vi "stringsubsect.vi"() -> ()   [LabVIEW 2019]
panel:
  out "substring":string
  in  "String":string
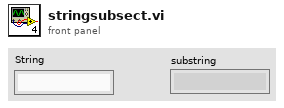
[diagram p1: front panel]
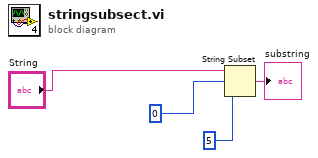
[diagram p0: block diagram]
diagram:
  n1 = String Subset(string="String", offset (0)=0, length (rest)=5 ("length (rest)")) -> (substring=→"substring":string)
